vi "Agilent VNA Convert 8510 Status Bytes.vi"(2 "8510 Status Bytes":bool[](array[boolean])=[FALSE, FALSE, FALSE, FALSE, FALSE, FALSE, FALSE, FALSE, FALSE, FALSE, FALSE, FALSE, FALSE, FALSE, FALSE, FALSE, FALSE, FALSE, FALSE, FALSE, FALSE, FALSE, FALSE, FALSE, FALSE, FALSE, FALSE, FALSE, FALSE, FALSE, FALSE, FALSE]) -> (6 "Event Status Register B":bool[](array[boolean]), 7 "Event Status Register":bool[](array[boolean]))   [LabVIEW 2011]
panel:
  # "Caution Message Displayed\n\nData Entry Complete\n\nTRIG Mode\n\nOne-path-2-port Measurement\n\nOperation Complete\n\nSyntax Error\n\nRQS Issued\n\nReason in Extened Byte\n\nNOT USED\n\nKey Pressed\n\nPower On Sequence Complete\n\nNOT USED\n\nNOT USED\n\nNOT USED\n\nNOT USED\n\nNOT USED"
  # "Single, Num of Groups, or Cal Standard Complete\n\nService Routine Waiting\n\nData Entry Complete\n\nLimit Failed CH 2\n\nLimit Failed CH 1\n\nSearch Fail CH 2\n\nSearch Fail CH 1\n\nALC Unlock"
  # "Operation Complete\n\nRequest Control\n\nQuery Error\n\n\n\nExecution Error\n\nSyntax Error (GP-IB)\n\nUser Request\n\nPower On"
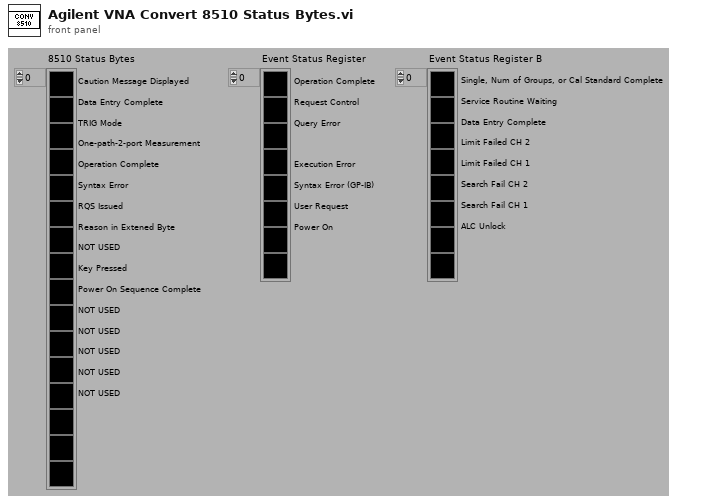
[diagram p1: front panel]
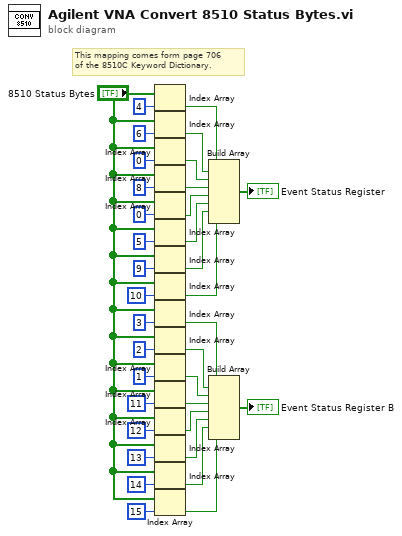
[diagram p0: block diagram]
diagram:
  # "This mapping comes form page 706\nof the 8510C Keyword Dictionary."
  n1 = Index Array(array="8510 Status Bytes", index=4) -> (element=w19:bool)
  n2 = Index Array(array="8510 Status Bytes", index=6) -> (element=w10:bool)
  n3 = Index Array(array="8510 Status Bytes", index=0) -> (element=w9:bool)
  n4 = Index Array(array="8510 Status Bytes", index=8) -> (element=w18:bool)
  n5 = Index Array(array="8510 Status Bytes", index=0) -> (element=w11:bool)
  n6 = Index Array(array="8510 Status Bytes", index=5) -> (element=w12:bool)
  n7 = Index Array(array="8510 Status Bytes", index=9) -> (element=w13:bool)
  n8 = Index Array(array="8510 Status Bytes", index=10) -> (element=w16:bool)
  n9 = Index Array(array="8510 Status Bytes", index=3) -> (element=w15:bool)
  n10 = Index Array(array="8510 Status Bytes", index=2) -> (element=w3:bool)
  n11 = Index Array(array="8510 Status Bytes", index=1) -> (element=w2:bool)
  n12 = Index Array(array="8510 Status Bytes", index=11) -> (element=w14:bool)
  n13 = Index Array(array="8510 Status Bytes", index=12) -> (element=w7:bool)
  n14 = Index Array(array="8510 Status Bytes", index=13) -> (element=w4:bool)
  n15 = Index Array(array="8510 Status Bytes", index=14) -> (element=w5:bool)
  n16 = Index Array(array="8510 Status Bytes", index=15) -> (element=w6:bool)
  n17 = Build Array(w19, w10, w9, w18, w11, w12, w13, w16) -> (→"Event Status Register":bool[])
  n18 = Build Array(w15, w3, w2, w14, w7, w4, w5, w6) -> (→"Event Status Register B":bool[])
